vi "New Maze.vi"(8 "error in (no error)":errorcluster, 10 "Maze Level":T1, 11 "Mouse in":refnum<class "Mouse.lvclass">) -> (0 "error out":errorcluster, 3 "Mouse out":refnum<class "Mouse.lvclass">)   [LabVIEW 2020, in "Maze.lvlib" / "Mouse.lvclass"]
doc: "New Maze is called whenever the current maze is changed so that the mouse can reset its memory if necessary since the same maze wont be run again. When this VI is called the new maze's difficulty level is specified incase the mouse uses an optimized algorithm for each maze level."
uses:
  Mouse.lvclass
  Maze Level.ctl
  Maze.lvlib
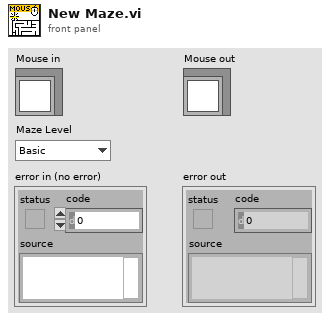
[diagram p1: front panel]
types:
  T1 = typedef "Maze.lvlib/Maze Level.ctl" = enum16{"Basic", "Intermediate", "Advanced", "Quantum"}
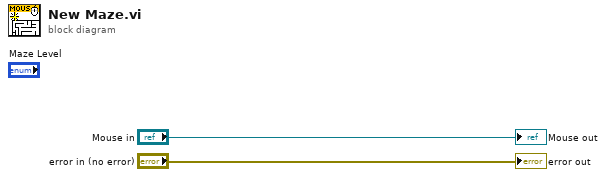
[diagram p0: block diagram]
diagram:
  "error out" <- "error in (no error)"
  "Mouse out" <- "Mouse in"
